vi "TestMain - Log - TDMS v2.vi"() -> ()   [LabVIEW 2019]
uses:
  <vilib>/myRIO/Instrument Drivers/Onboard IO/I2C/typedefs/I2C User Configuration.ctl
  <vilib>/myRIO/Instrument Drivers/Onboard IO/I2C/typedefs/I2C Transfer Rate.ctl
  <vilib>/Platform/TimedLoop/XDataNode/timing_clust.ctl
  <vilib>/Platform/TimedLoop/XDataNode/nitl_modes.ctl
  <vilib>/Platform/TimedLoop/XDataNode/wakeup.ctl
  <vilib>/userdefined/High Color/nirio_resource_hc.ctl
  <vilib>/myRIO/Instrument Drivers/Onboard IO/PWM/typedefs/PWM Reference.ctl
  <vilib>/myRIO/Common/Instrument Driver Framework/Utilities/typedefs/myRIO Generic Hardware Reference.ctl
  <vilib>/myRIO/Common/Instrument Driver Framework/Utilities/typedefs/Hardware Version Enum.ctl
  <vilib>/myRIO/Common/Instrument Driver Framework/Utilities/typedefs/myRIO v1.0 Reference.ctl
  <vilib>/myRIO/Common/Instrument Driver Framework/Utilities/typedefs/Generic FPGA Reference.ctl
  <vilib>/myRIO/Common/Instrument Driver Framework/myRIO v1.0/PWM/typedefs/PWM Channels Enum.ctl
  <vilib>/myRIO/Instrument Drivers/Onboard IO/PWM/typedefs/PWM Configuration.ctl
  <vilib>/myRIO/Instrument Drivers/Onboard IO/DIO/typedefs/DIO Reference.ctl
  <vilib>/myRIO/Common/Instrument Driver Framework/myRIO v1.0/DIO/typedefs/DIO Channels List.ctl
  <vilib>/myRIO/Common/Instrument Driver Framework/myRIO v1.0/DIO/typedefs/DIO Channels Enum.ctl
  <vilib>/myRIO/Common/Instrument Driver Framework/Utilities/vis/Is FPGA Ref Available.vi
  <vilib>/myRIO/Common/Instrument Driver Framework/myRIO v1.0/PWM/vis/myRIO v1.1 Open PWM.vi
  <vilib>/myRIO/Instrument Drivers/Onboard IO/PWM/vis/Set Duty Cycle and Frequency.vi
  <vilib>/myRIO/Common/Instrument Driver Framework/myRIO v1.0/DIO/vis/myRIO v1.1 Open DIO.vi
  <extravilib>/ChannelInstances/Tag-bool/Write With Abort.vi
  <extravilib>/ChannelInstances/Tag-bool/Read With Abort.vi
  <vilib>/myRIO/Common/Instrument Driver Framework/myRIO v1.0/I2C/vis/myRIO v1.0 Close I2C.vi
  <vilib>/myRIO/Common/Instrument Driver Framework/Utilities/vis/Validate Channels.vi
  <vilib>/myRIO/Common/Instrument Driver Framework/myRIO v1.0/PWM/vis/myRIO v1.0 Reserve PWM.vi
  <vilib>/myRIO/Common/Instrument Driver Framework/myRIO v1.0/DIO/vis/myRIO v1.0 Reserve DIO.vi
  <vilib>/myRIO/Common/Instrument Driver Framework/myRIO v1.0/UART/vis/myRIO v1.0 Close UART.vi
  <vilib>/myRIO/Common/Instrument Driver Framework/myRIO v1.0/I2C/vis/myRIO v1.0 Unreserve I2C.vi
  <vilib>/myRIO/Common/Instrument Driver Framework/myRIO v1.0/PWM/vis/myRIO v1.0 Build MUX Configuration PWM.vi
  <vilib>/myRIO/Common/Instrument Driver Framework/myRIO v1.0/Resource Manager/vis/myRIO v1.0 Reserve Channel List.vi
  <vilib>/myRIO/Common/Instrument Driver Framework/myRIO v1.0/DIO/vis/myRIO v1.0 Build MUX Configuration DIO.vi
  <vilib>/myRIO/Common/Instrument Driver Framework/myRIO v1.0/I2C/vis/myRIO v1.0 Build MUX Configuration I2C.vi
  <vilib>/myRIO/Common/Instrument Driver Framework/myRIO v1.0/Resource Manager/vis/myRIO v1.0 Unreserve Channel List.vi
  <vilib>/myRIO/Common/Instrument Driver Framework/myRIO v1.0/Resource Manager/vis/myRIO v1.0 Create Configuration List.vi
  <vilib>/myRIO/Common/Instrument Driver Framework/myRIO v1.0/Resource Manager/vis/myRIO v1.0 Reserve Channel.vi
  <vilib>/myRIO/Common/Instrument Driver Framework/myRIO v1.0/Resource Manager/vis/myRIO v1.0 Unreserve Channel.vi
  <vilib>/myRIO/Common/Instrument Driver Framework/myRIO v1.0/Resource Manager/vis/myRIO v1.0 Build Mutex Name.vi
  <vilib>/FPGAPlugInAG/myRIO-1900/niLvFpga_Open_myRIO-1900.vi
  <vilib>/rvi/interface/common/dynamic/niFpgaDynamicAddResources.vi
  <vilib>/Utility/error.llb/Error Cluster From Error Code.vi
  <vilib>/rvi/errors/niLvFpgaAdjustHostInterfaceError.vi
  <vilib>/myRIO/Common/Instrument Driver Framework/Utilities/vis/FPGA Ref Manager.vi
  <vilib>/myRIO/Common/Instrument Driver Framework/Utilities/vis/Ref Counter.vi
  <vilib>/FPGAPlugInAG/Dynamic/niLvFpga_Run_Dynamic.vi
  <vilib>/myRIO/Common/Instrument Driver Framework/myRIO v1.0/I2C/vis/myRIO v1.0 Configure I2C.vi
  <vilib>/myRIO/Common/Instrument Driver Framework/myRIO v1.0/I2C/vis/myRIO v1.0 Write I2C.vi
  <vilib>/Utility/VariantDataType/GetNumericInfo.vi
  <vilib>/myRIO/Common/Instrument Driver Framework/myRIO v1.0/myRIO v1.1 Open.vi
  <vilib>/myRIO/Common/Instrument Driver Framework/Utilities/vis/IO Manager.vi
  <vilib>/myRIO/Common/Instrument Driver Framework/Utilities/vis/Configuration Manager.vi
  <vilib>/myRIO/Common/Instrument Driver Framework/myRIO v1.0/Resource Manager/vis/myRIO v1.0 Configure IO.vi
  <vilib>/myRIO/Common/Instrument Driver Framework/myRIO v1.0/myRIO v1.0 Close.vi
  <vilib>/myRIO/Common/Instrument Driver Framework/myRIO v1.0/PWM/vis/myRIO v1.0 Write PWM.vi
  <vilib>/myRIO/Common/Instrument Driver Framework/myRIO v1.0/DIO/vis/myRIO v1.0 Write DIO.vi
  <vilib>/Instr/_visa.llb/VISA Configure Serial Port (Instr).vi
  <extravilib>/ChannelInstances/Tag-bool/Instantiate.vi
  <extravilib>/ChannelInstances/Tag-bool/EndpointRead.vi
  <vilib>/myRIO/Common/Instrument Driver Framework/myRIO v1.0/I2C/vis/myRIO v1.0 Read I2C.vi
  <vilib>/myRIO/Common/Instrument Driver Framework/myRIO v1.0/I2C/vis/myRIO v1.0 Shutdown I2C.vi
  <vilib>/FPGAPlugInAG/Dynamic/niLvFpga_Abort_Dynamic.vi
  <vilib>/myRIO/Common/Instrument Driver Framework/myRIO v1.0/myRIO v1.0 Reset FPGA.vi
  <vilib>/myRIO/Common/Instrument Driver Framework/myRIO v1.0/IRQ/vis/myRIO v1.0 IRQ Info FGV.vi
  <vilib>/myRIO/Common/Instrument Driver Framework/myRIO v1.0/IRQ/vis/myRIO v1.0 Timer IRQ Info FGV.vi
  <vilib>/myRIO/Common/Instrument Driver Framework/myRIO v1.0/IRQ/vis/myRIO v1.0 ISR Agent.vi
  <vilib>/myRIO/Instrument Drivers/Utilities/vis/Reset Index.vi
  <vilib>/myRIO/Common/Instrument Driver Framework/myRIO v1.0/Resource Manager/vis/myRIO v1.0 Block Write Resource Manager.vi
  <vilib>/FPGAPlugInAG/Dynamic/niLvFpga_Close_Dynamic.vi
  <extravilib>/ChannelInstances/Tag-bool/Endpoint.vi
  <vilib>/platform/TimedLoop/XDataNode/XDataNode.xnode
  <vilib>/rvi/interface/nirviOpenFPGA/nirviOpenFPGA.xnode
  Documents/Source_Distribution/AutoBike_Autumn2021_src_lvproj/home/lvuser/natinst/bin/autobike_FPGATarget_myRIO-1900Custom_zQgCF+RzkZg.lvbitx
  <vilib>/rvi/interface/nirviReadWriteControl/nirviReadWriteControl.xnode
  <vilib>/rvi/interface/nirviMethod/nirviMethod.xnode
  <vilib>/myRIO/Express VI/Onboard IO/PWM/PWM Express VI.xnode
  <vilib>/myRIO/Instrument Drivers/Onboard IO/PWM/vis/myRIO PWM Open.xnode
  <vilib>/myRIO/Express VI/Onboard IO/DO/DO Express VI.xnode
  <vilib>/myRIO/Instrument Drivers/Onboard IO/DIO/vis/myRIO DIO Open.xnode
  <vilib>/rvi/interface/nirviCloseFPGA/nirviCloseFPGA.xnode
  <vilib>/myRIO/Instrument Drivers/Utilities/Utilities.lvlib
  NiFpgaLv.dll
  <vilib>/rvi/interface/Simulation/niFpgaSimulationCallBeginRW.vi
  <vilib>/Platform/TimedLoop/XDataNode/XDNodeRunTimeDep.lvlib
  <extravilib>/ChannelInstances/Tag-bool.lvlib
  <vilib>/myRIO/Instrument Drivers/Onboard IO/I2C/I2C.lvlib
  <vilib>/myRIO/Instrument Drivers/Onboard IO/DIO/DIO.lvlib
  <vilib>/myRIO/Instrument Drivers/Onboard IO/PWM/PWM.lvlib
panel:
  out "Raw output from GPS":string
  in  "Organised Output from the GPS":T1(tab)
  out "GPGSV":string
  out "number of message":string
  out "msg1":string
  out "Satelite in view":string
  in  "Satelite_id/elevation/azimuth/SNR 17":enum32{"Msg 1", "Msg 2", "Msg 3", "Msg 4"}(tab)
  out "Satelite_id/elevation/azimuth/SNR":string[](array[string])
  out "Satelite_id/elevation/azimuth/SNR 2":string[](array[string])
  out "Satelite_id/elevation/azimuth/SNR 3":string[](array[string])
  out "Satelite_id/elevation/azimuth/SNR 4":string[](array[string])
  out "Signal ID / Check sum":string[](array[string])
  out "Signal ID / Check sum 2":string[](array[string])
  out "Satelite_id/elevation/azimuth/SNR 8":string[](array[string])
  out "Satelite_id/elevation/azimuth/SNR 7":string[](array[string])
  out "Satelite_id/elevation/azimuth/SNR 6":string[](array[string])
  out "Satelite_id/elevation/azimuth/SNR 5":string[](array[string])
  out "Signal ID / Check sum 3":string[](array[string])
  out "Satelite_id/elevation/azimuth/SNR 12":string[](array[string])
  out "Satelite_id/elevation/azimuth/SNR 11":string[](array[string])
  out "Satelite_id/elevation/azimuth/SNR 10":string[](array[string])
  out "Satelite_id/elevation/azimuth/SNR 9":string[](array[string])
  out "Signal ID / Check sum 4":string[](array[string])
  out "Satelite_id/elevation/azimuth/SNR 16":string[](array[string])
  out "Satelite_id/elevation/azimuth/SNR 15":string[](array[string])
  out "Satelite_id/elevation/azimuth/SNR 14":string[](array[string])
  out "Satelite_id/elevation/azimuth/SNR 13":string[](array[string])
  out "GLGSV 2":string
  out "number of message 2":string
  out "msg1 2":string
  out "Satelite in view 2":string
  in  "Satelite_id/elevation/azimuth/SNR 34":enum32{"Msg 1", "Msg 2", "Msg 3", "Msg 4"}(tab)
  out "Satelite_id/elevation/azimuth/SNR 21":string[](array[string])
  out "Satelite_id/elevation/azimuth/SNR 20":string[](array[string])
  out "Satelite_id/elevation/azimuth/SNR 19":string[](array[string])
  out "Satelite_id/elevation/azimuth/SNR 18":string[](array[string])
  out "Signal ID / Check sum 5":string[](array[string])
  out "Signal ID / Check sum 6":string[](array[string])
  out "Satelite_id/elevation/azimuth/SNR 25":string[](array[string])
  out "Satelite_id/elevation/azimuth/SNR 22":string[](array[string])
  out "Satelite_id/elevation/azimuth/SNR 23":string[](array[string])
  out "Satelite_id/elevation/azimuth/SNR 24":string[](array[string])
  out "Signal ID / Check sum 7":string[](array[string])
  out "Satelite_id/elevation/azimuth/SNR 29":string[](array[string])
  out "Satelite_id/elevation/azimuth/SNR 26":string[](array[string])
  out "Satelite_id/elevation/azimuth/SNR 27":string[](array[string])
  out "Satelite_id/elevation/azimuth/SNR 28":string[](array[string])
  out "Signal ID / Check sum 8":string[](array[string])
  out "Satelite_id/elevation/azimuth/SNR 33":string[](array[string])
  out "Satelite_id/elevation/azimuth/SNR 30":string[](array[string])
  out "Satelite_id/elevation/azimuth/SNR 31":string[](array[string])
  out "Satelite_id/elevation/azimuth/SNR 32":string[](array[string])
  out "GAGSV 3":string
  out "number of message 3":string
  out "msg1 3":string
  out "Satelite in view 3":string
  in  "Satelite_id/elevation/azimuth/SNR 51":enum32{"Msg 1", "Msg 2", "Msg 3", "Msg 4"}(tab)
  out "Satelite_id/elevation/azimuth/SNR 38":string[](array[string])
  out "Satelite_id/elevation/azimuth/SNR 37":string[](array[string])
  out "Satelite_id/elevation/azimuth/SNR 36":string[](array[string])
  out "Satelite_id/elevation/azimuth/SNR 35":string[](array[string])
  out "Signal ID / Check sum 9":string[](array[string])
  out "Signal ID / Check sum 10":string[](array[string])
  out "Satelite_id/elevation/azimuth/SNR 42":string[](array[string])
  out "Satelite_id/elevation/azimuth/SNR 39":string[](array[string])
  out "Satelite_id/elevation/azimuth/SNR 40":string[](array[string])
  out "Satelite_id/elevation/azimuth/SNR 41":string[](array[string])
  out "Signal ID / Check sum 11":string[](array[string])
  out "Satelite_id/elevation/azimuth/SNR 46":string[](array[string])
  out "Satelite_id/elevation/azimuth/SNR 43":string[](array[string])
  out "Satelite_id/elevation/azimuth/SNR 44":string[](array[string])
  out "Satelite_id/elevation/azimuth/SNR 45":string[](array[string])
  out "Signal ID / Check sum 12":string[](array[string])
  out "Satelite_id/elevation/azimuth/SNR 50":string[](array[string])
  out "Satelite_id/elevation/azimuth/SNR 47":string[](array[string])
  out "Satelite_id/elevation/azimuth/SNR 48":string[](array[string])
  out "Satelite_id/elevation/azimuth/SNR 49":string[](array[string])
  out "GBGSV 4":string
  out "number of message 4":string
  out "msg1 4":string
  out "Satelite in view 4":string
  in  "Satelite_id/elevation/azimuth/SNR 68":enum32{"Msg 1", "Msg 2", "Msg 3", "Msg 4"}(tab)
  out "Satelite_id/elevation/azimuth/SNR 55":string[](array[string])
  out "Satelite_id/elevation/azimuth/SNR 54":string[](array[string])
  out "Satelite_id/elevation/azimuth/SNR 53":string[](array[string])
  out "Satelite_id/elevation/azimuth/SNR 52":string[](array[string])
  out "Signal ID / Check sum 13":string[](array[string])
  out "Signal ID / Check sum 14":string[](array[string])
  out "Satelite_id/elevation/azimuth/SNR 59":string[](array[string])
  out "Satelite_id/elevation/azimuth/SNR 56":string[](array[string])
  out "Satelite_id/elevation/azimuth/SNR 57":string[](array[string])
  out "Satelite_id/elevation/azimuth/SNR 58":string[](array[string])
  out "Signal ID / Check sum 15":string[](array[string])
  out "Satelite_id/elevation/azimuth/SNR 63":string[](array[string])
  out "Satelite_id/elevation/azimuth/SNR 60":string[](array[string])
  out "Satelite_id/elevation/azimuth/SNR 61":string[](array[string])
  out "Satelite_id/elevation/azimuth/SNR 62":string[](array[string])
  out "Signal ID / Check sum 16":string[](array[string])
  out "Satelite_id/elevation/azimuth/SNR 67":string[](array[string])
  out "Satelite_id/elevation/azimuth/SNR 64":string[](array[string])
  out "Satelite_id/elevation/azimuth/SNR 65":string[](array[string])
  out "Satelite_id/elevation/azimuth/SNR 66":string[](array[string])
  out "UTC Time":string
  out "N/S":string
  out "Long":string
  out "Mode":string
  out "Status":string
  out "Lat":string
  out "Course over Ground [Degrees]":string
  out "date[ddmmyy]":string
  out "E/W":string
  out "Speed over ground[knot]":string
  out "xxRMC":string
  out "NavStatus":string
  out "Checksum":string
  out "Carriage return":string
  out "Lat 2":string
  out "NS":string
  out "GLL":string
  out "Long 3":string
  out "EW":string
  out "Time":string
  out "Status 2":string
  out "Positioning mod":string
  out "Check sum":string
  out "Carriage return 2":string
  out "VTG":string
  out "Course over Ground":string
  out "Reference":string
  out "Course over Ground (Magnetic)":string
  out "Reference2":string
  out "Speedover Ground (knots)":string
  out "Units1":string
  out "Speed over ground kph":string
  out "Units 2":string
  out "Position Mode 2":string
  out "Check sum 2":string
  out "GGA 3":string
  out "UTC time":string
  out "Lat 3":string
  out "NS 2":string
  out "Long 2":string
  out "EW 2":string
  out "Pos_indicator":string
  out "Number of Satelite_used":string
  out "hdop":string
  out "msl_altitude":string
  out "altitude_units":string
  out "geoidal_Seperation":string
  out "Separation unit":string
  out "age of Diff corr":string
  out "diffStating":string
  out "Checksum 2":string
  out "GSA":string
  out "Operation Mode":string
  out "Navigation mode":string
  out "satelite used channel 1":string
  out "satelite used channel 3":string
  out "satelite used channel 4":string
  out "satelite used channel 5":string
  out "satelite used channel 6":string
  out "satelite used channel 7":string
  out "satelite used channel 8":string
  out "satelite used channel 9":string
  out "satelite used channel 10":string
  out "satelite used channel 11":string
  out "satelite used channel 12":string
  out "pdop":string
  out "hdop 2":string
  out "vdop":string
  out "System ID":string
  out "Checksum 3":string
  out "satelite used channel 2":string
  in  "Name of the Logging file":string="Logging.tdms"
  out "Path to the Logg file":path
  out "Combined duration time (us)":i64
  in  "Loop durations":T2(tab)
  out "IMU Data gathering duration(us)":i64(graph)
  out "Hall data gathering duration(us)":i64(graph)
  out "Encoder data gathering duration(us)":i64(graph)
  out "Steering Motor Sending/updating value duration(us)":i64(graph)
  out "E-Stop loop duration (us)":i64(graph)
  out "GPS loop duration (us)":i64(graph)
  in  "Duty cycle":dbl(slide)=0.5 step=0.01 scale=0.1..0.9
  in  "GO":bool
  out "E-Stop":bool
  in  "E-stop":bool
  in  "IMU":bool
  out "IMU Acc Chart":cluster{dbl, dbl, dbl}(graph)
  out "IMU Gyro Chart":cluster{dbl, dbl, dbl}(graph)
  out "Encoder Position (Counts)":i32
  out "Encoder Acceleration (Counts/Interval)":i32
  out "Encoder Velocity (Counts/Interval)":i32
  in  "Encoder":bool
  in  "Encoder Position Reset":bool
  out "Hall Period":u32
  in  "Hall":bool
  out "Hall Detection":bool
  # "Signal ID / Check sum"
  # "Signal ID / Check sum"
  # "Signal ID / Check sum"
  # "Signal ID / Check sum"
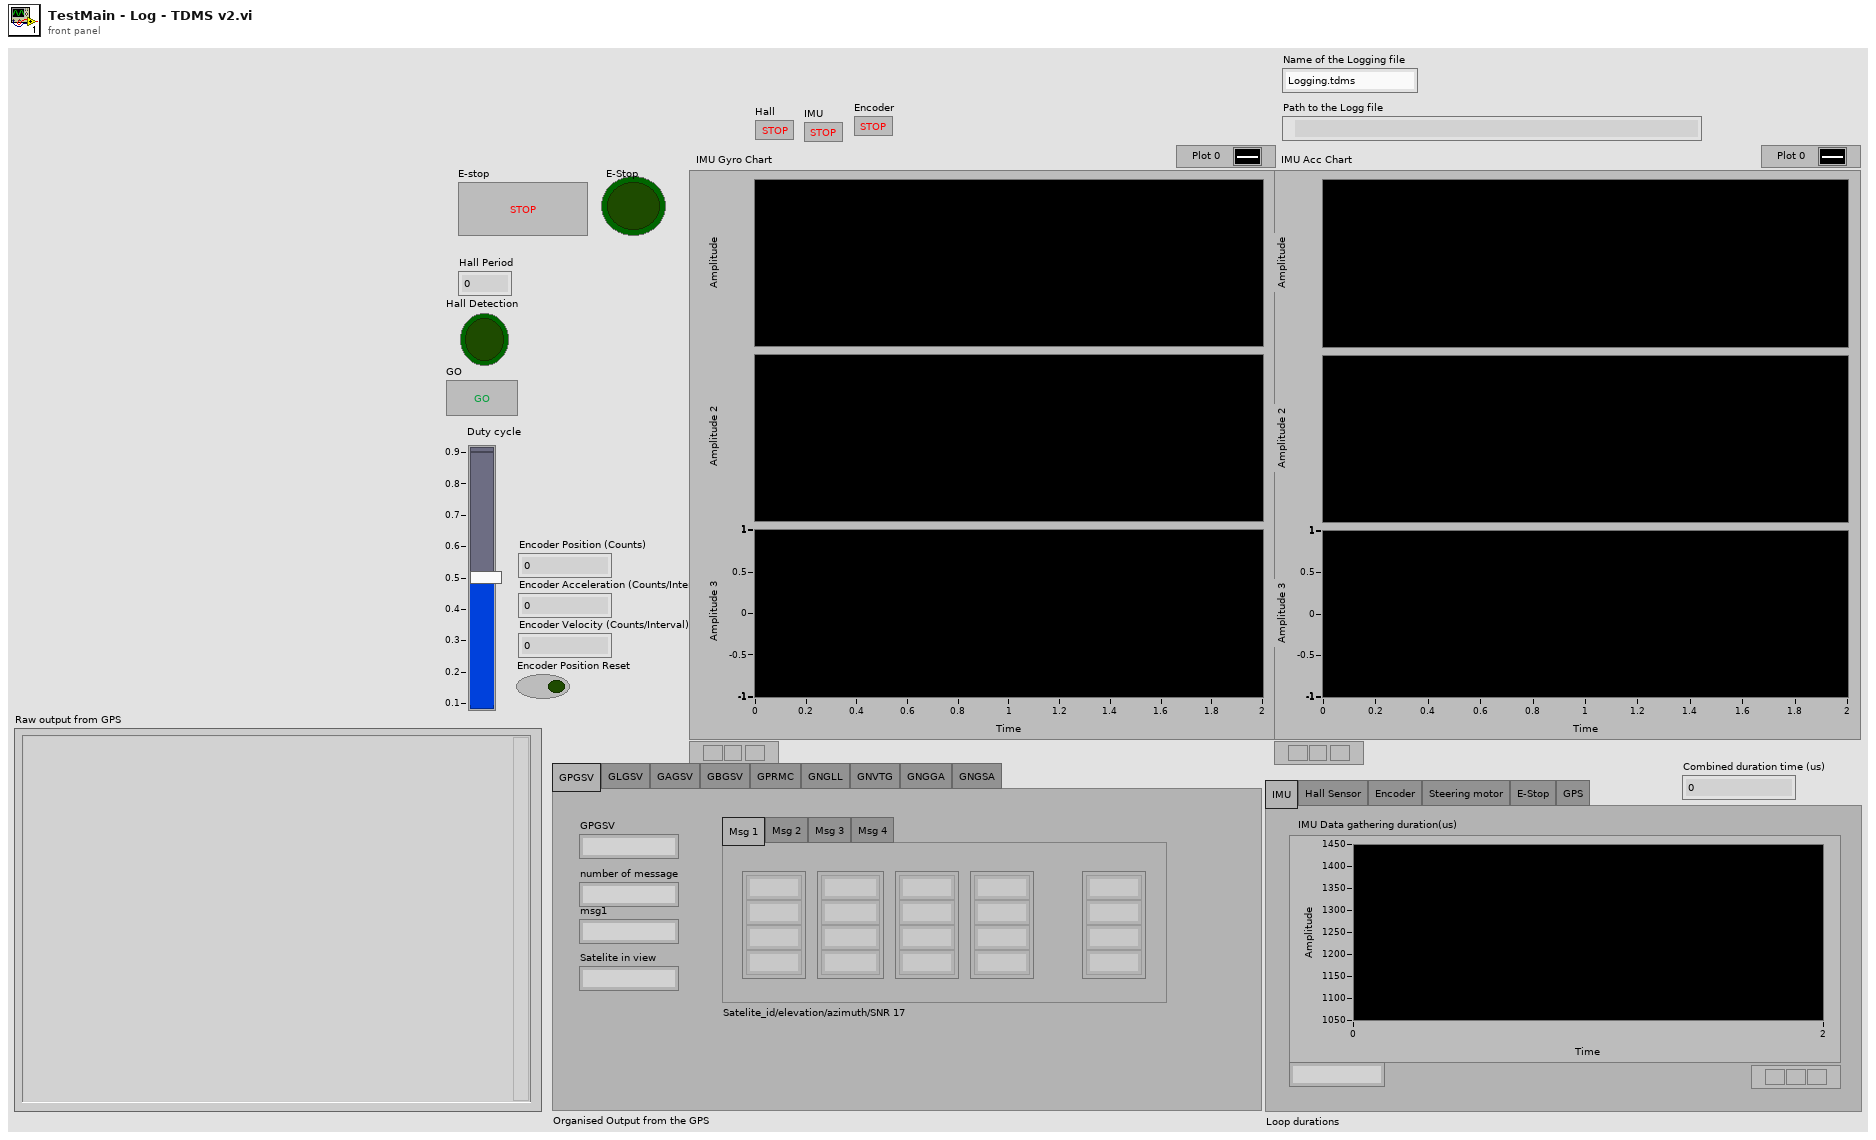
[diagram p1: front panel]
types:
  T1 = enum32{"GPGSV", "GLGSV", "GAGSV", "GBGSV", "GPRMC", "GNGLL", "GNVTG", "GNGGA", "GNGSA"}
  T2 = enum32{"IMU", "Hall Sensor", "Encoder", "Steering motor", "E-Stop", "GPS"}
  T3 = typedef "I2C.lvlib/I2C User Configuration.ctl" = cluster{"I2C Transfer Rate":T4}
  T4 = typedef "I2C.lvlib/I2C Transfer Rate.ctl" = enum16{"Standard mode (100 kbps)", "Fast mode (400 kbps)"}
  T5 = enum16{"open", "open or create", "create or replace", "create", "open (read-only)"}
  T6 = typedef "nirio_resource_hc.ctl" = tag
  T7 = typedef "I2C.lvlib/I2C Reference.ctl" = cluster{"myRIO Reference":T8, "I2C Channels Enum":T12, "I2C Configuration":T13}
  T8 = typedef "myRIO Generic Hardware Reference.ctl" = cluster{"myRIO Model":T9, "myRIO Hardware Reference":T10}
  T9 = typedef "Hardware Version Enum.ctl" = enum16{"Unknown", "myRIO-1900", "myRIO-1950", "roboRIO", "NI ELVIS RIO CM", "ELVIS III"}
  T10 = typedef "myRIO v1.0 Reference.ctl" = cluster{"Generic FPGA Reference":T11, "Allow multiple opens":bool}
  T11 = typedef "Generic FPGA Reference.ctl" = refnum<k20>
  T12 = typedef "I2C Channels Enum.ctl" = enum16{"Not Connected", "A/I2C", "B/I2C", "I2C/I2C"}
  T13 = typedef "I2C.lvlib/I2C Configuration.ctl" = cluster{"I2C Transfer Rate":T4}
  T14 = typedef "XDNodeRunTimeDep.lvlib/timing_clust.ctl" = cluster{"Expected End [f-1]":u64, "Actual End [f-1]":u64, "Finished Late? [f-1]":bool, "Expected End [i-1]":u64, "Actual End [i-1]":u64, "Finished Late? [i-1]":bool, "Expected Start [i]":u64, "Actual Start [i]":u64, "Expected Start [f]":u64, "Actual Start [f]":u64, "Source Name":string, "Structure Name":string, "Period":i64, "Deadline":i64, "Offset":i64, "Start":i64, "Priority":i32, "Timeout":i32, "Mode":T15, "Wakeup Reason":T16, "Error":errorcluster, "Source Type":string, "Secondary Source Type":string, "Global End Time":u64, "Global Start Time":u64, "Frame Duration":u64, "Iteration Duration":u64, "Assigned CPU":i32, "I/O Scan Engine Mode":u32}
  T15 = typedef "XDNodeRunTimeDep.lvlib/nitl_modes.ctl" = enum32{"No Change", "Process missed periods, maintain original phase", "Discard missed periods, maintain original phase", "Process missed periods, ignore original phase", "Discard missed periods, ignore original phase"}
  T16 = typedef "XDNodeRunTimeDep.lvlib/wakeup.ctl" = enum32{"Normal", "Aborted", "Asynchronous wakeup", "Timing source error", "Timed loop error", "Timeout"}
  T17 = typedef "PWM.lvlib/PWM Reference.ctl" = cluster{"myRIO Reference":T8, "PWM Channels Enum":T18, "PWM Configuration":T19}
  T18 = typedef "PWM Channels Enum.ctl" = enum16{"Not Connected", "C/PWM0", "C/PWM1", "A/PWM0", "A/PWM1", "A/PWM2", "A/PWM3", "A/PWM4", "A/PWM5", "A/PWM6", "A/PWM7", "A/PWM8", "A/PWM9", "A/PWM10", "A/PWM11", "A/PWM12", "A/PWM13", "A/PWM14", "A/PWM15", "A/PWM16", "A/PWM17", "A/PWM18", "A/PWM19", "B/PWM0", "B/PWM1", "B/PWM2", "B/PWM3", "B/PWM4", "B/PWM5", "B/PWM6", "B/PWM7", "B/PWM8", "B/PWM9", "B/PWM10", "B/PWM11", "B/PWM12", "B/PWM13", "B/PWM14", "B/PWM15", "B/PWM16", "B/PWM17", "B/PWM18", "B/PWM19", "PWM/PWM0", "PWM/PWM1", "PWM/PWM2", "PWM/PWM3", "PWM/PWM4", "PWM/PWM5", "PWM/PWM6", "PWM/PWM7", "PWM/PWM8", "PWM/PWM9"}
  T19 = typedef "PWM.lvlib/PWM Configuration.ctl" = cluster{"Frequency":dbl, "Duty Cycle":dbl}
  T20 = typedef "DIO.lvlib/DIO Reference.ctl" = cluster{"myRIO Reference":T8, "DIO Channels List":T21}
  T21 = typedef "DIO Channels List.ctl" = T22[]
  T22 = typedef "DIO Channels Enum.ctl" = enum16{"Not Connected", "C/DIO0", "C/DIO1", "C/DIO2", "C/DIO3", "C/DIO4", "C/DIO5", "C/DIO6", "C/DIO7", "A/DIO0", "A/DIO1", "A/DIO2", "A/DIO3", "A/DIO4", "A/DIO5", "A/DIO6", "A/DIO7", "A/DIO8", "A/DIO9", "A/DIO10", "A/DIO11", "A/DIO12", "A/DIO13", "A/DIO14", "A/DIO15", "A/DIO16", "A/DIO17", "A/DIO18", "A/DIO19", "B/DIO0", "B/DIO1", "B/DIO2", "B/DIO3", "B/DIO4", "B/DIO5", "B/DIO6", "B/DIO7", "B/DIO8", "B/DIO9", "B/DIO10", "B/DIO11", "B/DIO12", "B/DIO13", "B/DIO14", "B/DIO15", "B/DIO16", "B/DIO17", "B/DIO18", "B/DIO19", "LED0", "LED1", "LED2", "LED3", "Button0", "DIO/DIO0", "DIO/DIO1", "DIO/DIO2", "DIO/DIO3", "DIO/DIO4", "DIO/DIO5", "DIO/DIO6", "DIO/DIO7", "DIO/DIO8", "DIO/DIO9", "SPI/CS0", "SPI/CS1", "SPI/CS2", "SPI/CS3", "LED RADIO (Green)", "LED RADIO (Red)", "LED COMM (Green)", "LED COMM (Red)", "LED MODE (Green)", "LED MODE (Red)"}
  T23 = typedef "Tag-bool.lvlib/))Channel.ctl" = refnum<queue>
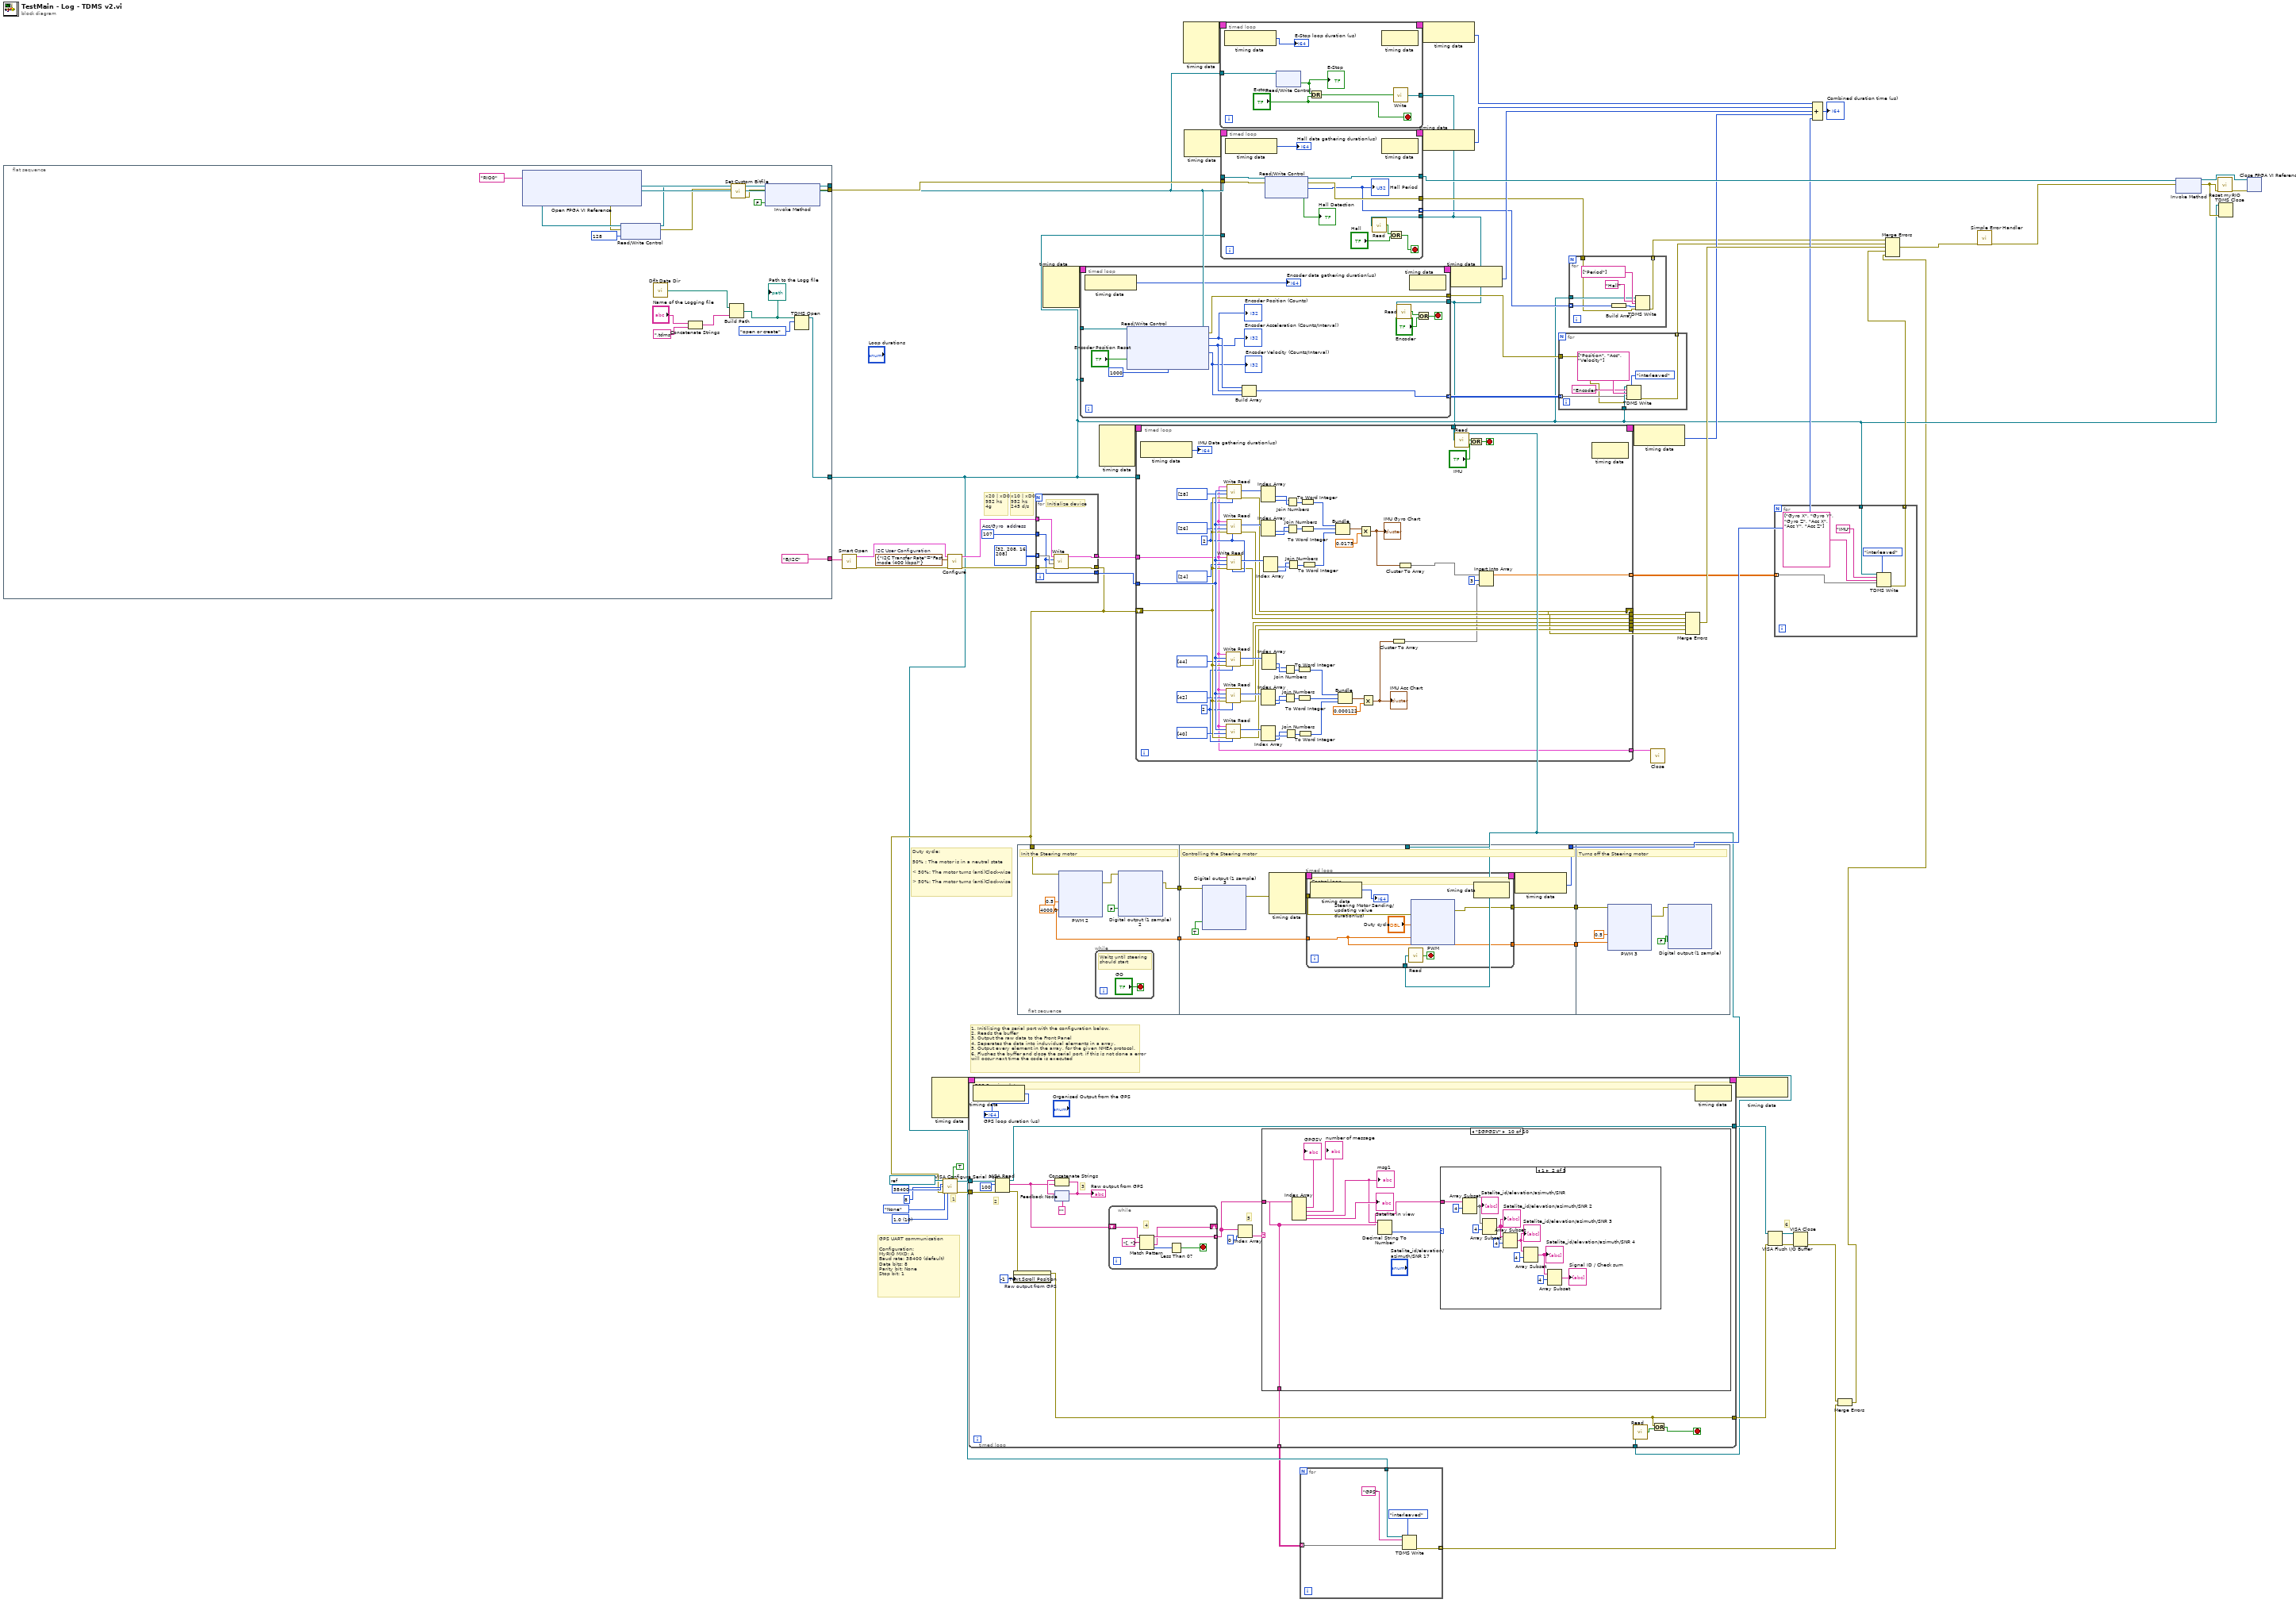
[diagram p0: block diagram]
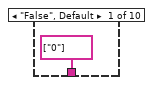
[diagram p2: hidden frame]
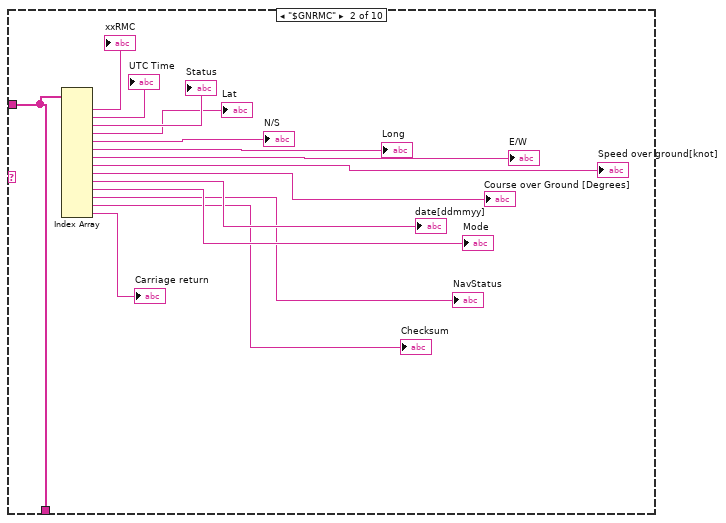
[diagram p3: hidden frame]
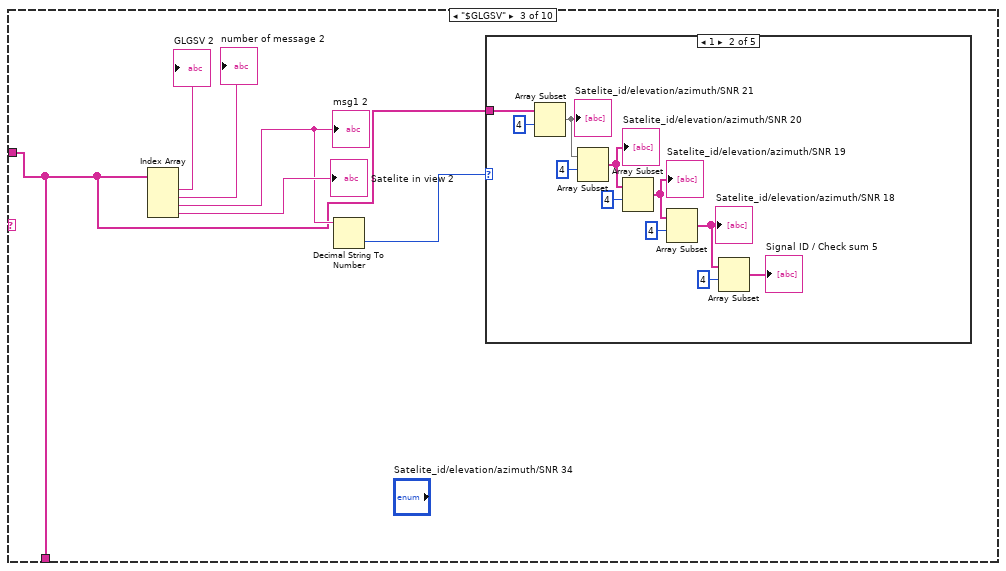
[diagram p4: hidden frame]
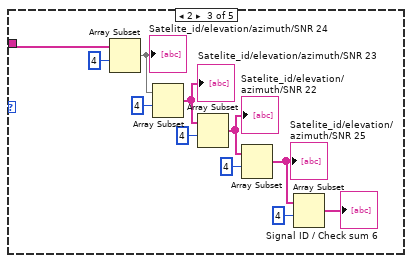
[diagram p6: hidden frame]
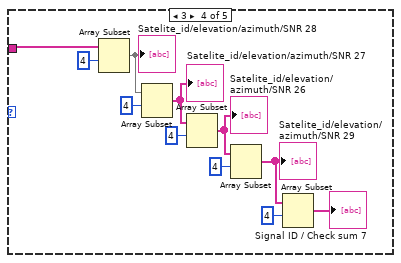
[diagram p7: hidden frame]
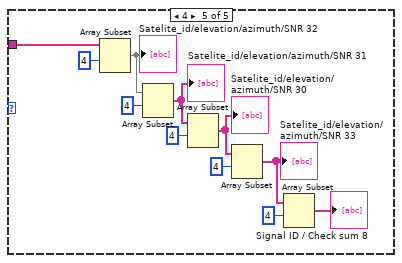
[diagram p8: hidden frame]
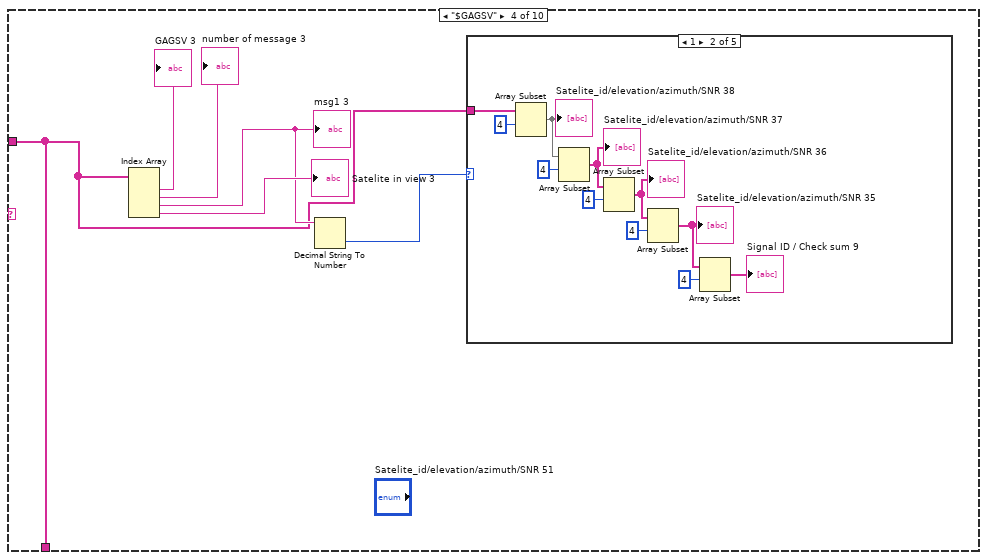
[diagram p9: hidden frame]
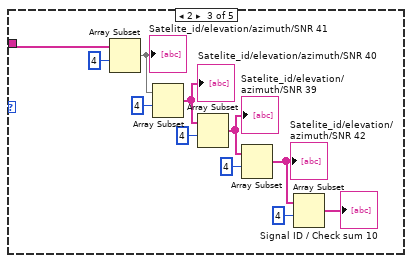
[diagram p11: hidden frame]
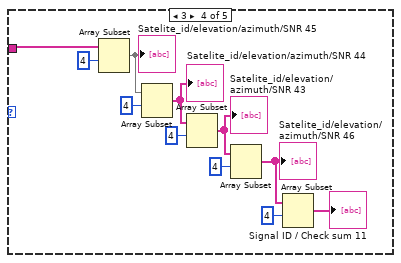
[diagram p12: hidden frame]
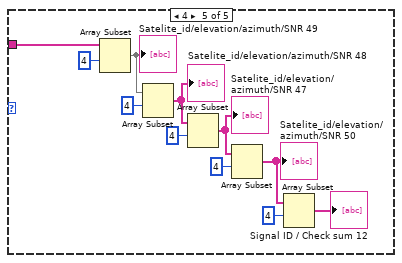
[diagram p13: hidden frame]
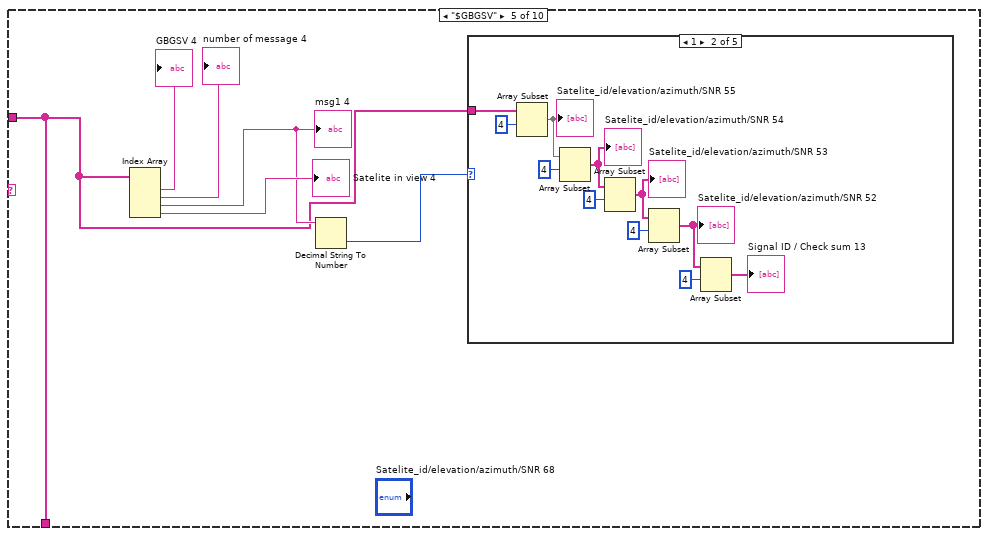
[diagram p14: hidden frame]
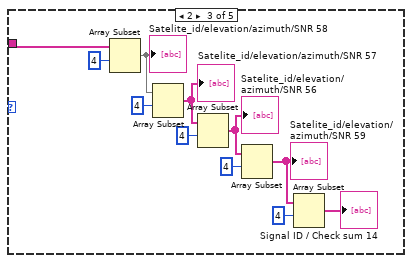
[diagram p16: hidden frame]
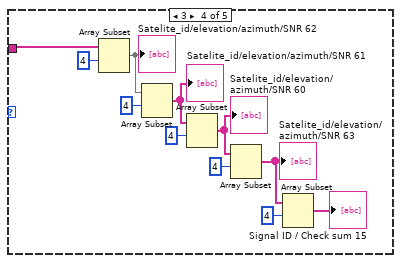
[diagram p17: hidden frame]
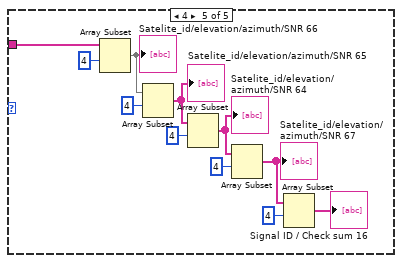
[diagram p18: hidden frame]
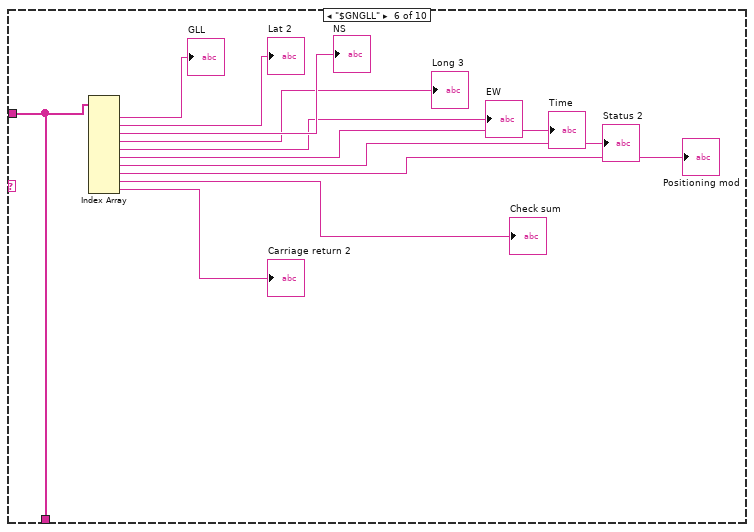
[diagram p19: hidden frame]
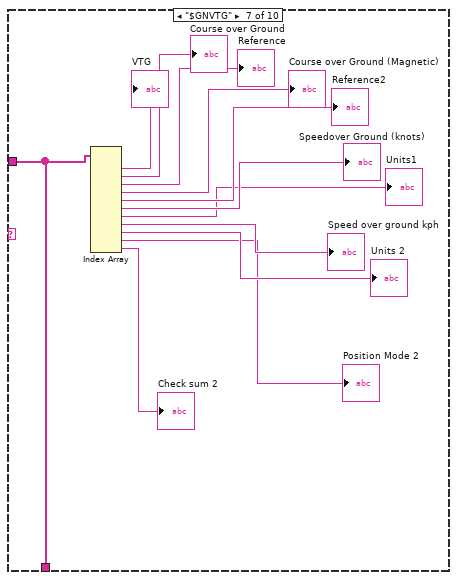
[diagram p20: hidden frame]
diagram:
  w15 = u16 10 items=["1.0"=10, "1.5"=15, "2.0"=20] ("stop bits (10: 1 bit)")
  w48 = u8 107  # Acc/Gyro  address
  w51 = T3 {"I2C Transfer Rate"=enum."Fast mode (400 kbps)"}  # I2C User Configuration
  # "6"
  # "1"
  # "1. Initilizing the serial port with the configuration below.\n2. Reads the buffer\n3. Output the raw data to the Front Panel\n4. Seperates the data into induvidual elements in a array.\n5. Output every element in the array, for the given NMEA protocol.\n6. Flushes the buffer and close the serial port, if this is not done a error will occur next time the code is executed"
  # "GPS UART communication\n\nConfiguration:\nMyRIO MXD: A\nBaud rate: 38400 (default)\nData bits: 8\nParity bit: None\nStop bit: 1"
  # "Duty cycle:\n\n50% : The motor is in a neutral state\n\n< 50%: The motor turns (anti)Clock-wise\n\n> 50%: The motor turns (anti)Clock-wise"
  # "x20 | xD0\n952 hz\n4g"
  # "x10 | xD0\n952 hz\n245 d/s"
  n1 = flat-sequence {
    tunnel: [w92] -> w61
    tunnel: [tag "B/I2C" ("I2C I/O")] -> w44
    tunnel: [w90] -> w40
    tunnel: [w80] -> w6
    frame #0 {
      n2 = xnode "Open FPGA VI Reference"("resource name"=T6 "RIO0" ("Resource name")) -> ("FPGA VI Reference Out"=w82:refnum<k20>, "error out"=w81:errorcluster)  [unwired: 1 in]
      n3 = xnode "Read/Write Control"("FPGA VI Reference In"=w82, "error in"=w81, "SYS.SELECTB"=u8 128) -> ("FPGA VI Reference Out"=w86:refnum<k20>, "error out"=w85:errorcluster)
      n4 = call <vilib>:"Dflt Data Dir.vi"() -> ("App:Default Data Directory"=w79:path)
      n5 = Concatenate Strings("Name of the Logging file", ".tdms" ("string")) -> (w74:string)
      n6 = Build Path(base path=w79, name or relative path=w74) -> (appended path=w78:path)
      "Path to the Logg file" <- w78
      n7 = call <vilib>:"Set Custom Bitfile.vi"("error in (no error)"=w85, "Custom FPGA Reference In"=w86) -> ("error out"=w87:errorcluster, "Custom FPGA Reference Out"=w89:refnum<k20>)  [unwired: 8 in]
      n8 = xnode "Invoke Method"("FPGA VI Reference In"=w89, "error in"=w87, "Wait Until Done (F)"=FALSE) -> ("FPGA VI Reference Out"=w90:refnum<k20>, "error out"=w92:errorcluster)
      n9 = TDMS Open(10:T5."open or create" ("operation (0:open)"), 11:w78) -> (3:w80:refnum<k34>)  [unwired: 5 in, 1 out]
    }
  }
  n10 = call <vilib>:"Smart Open.vi"("Channel Name"=w44) -> ("error out"=w49:errorcluster, "I2C Ref Out"=w50:T7)  [unwired: 9 in]
  n11 = node-c288() -> (w22:T14)  [unwired: 4 in]
  n12 = call <vilib>:"Configure.vi"("error in (no error)"=w49, "I2C User Configuration"=w51, "I2C Ref In"=w50) -> ("error out"=w45:errorcluster, "I2C Ref Out"=w46:T7)  [unwired: 7 in]
  n13 = flat-sequence {
    tunnel: [w97] -> w65
    tunnel: w8 -> [w95]
    tunnel: [w94] -> w64
    tunnel: w4 -> [w179]
    tunnel: w65 -> [w177]
    tunnel: w64 -> [w176]
    tunnel: [w175] -> w63
    tunnel: [w174] -> w62
    tunnel: [w171] -> w36
    tunnel: w63 -> [w266]
    tunnel: w62 -> [w265]
    frame #0 {
      w94 = 4000.0 ("Frequency [Hz]")
      # "Init the Steering motor"
      n14 = xnode "PWM 2"("Duty Cycle"=0.5, "Frequency [Hz]"=w94, "error in (no error)"=w95) -> ("error out"=w98:errorcluster)
      n15 = while {
        stop <- "GO" stop-if-true
        # "Waits until steering should start"
      }
      n16 = xnode "Digital output (1 sample) 2"("B/DIO4 (Pin 19)"=FALSE ("B/DIO1 (Pin 13)"), "error in (no error)"=w98) -> ("error out"=w97:errorcluster)
    }
    frame #1 {
      # "Controlling the Steering motor"
      n17 = xnode "Digital output (1 sample) 3"("B/DIO4 (Pin 19)"=TRUE ("B/DIO1 (Pin 13)"), "error in (no error)"=w177) -> ("error out"=w178:errorcluster)
      n18 = node-c288() -> (w173:T14)  [unwired: 4 in]
      n19 = timed-loop {
        tunnel: w179 -> [w184]
        tunnel: w178 -> [w183]
        tunnel: w176 -> [w182]
        tunnel: [w182] -> w175
        tunnel: [w181] -> w174
        timing: w173 -> [_]
        timing-out: [_] -> w172
        stop <- w185 stop-if-true
        # "Control loop"
        n20 = node-c288() -> (→"Steering Motor Sending/updating value duration(us)":i64)  [unwired: 1 in]
        n21 = call <extravilib>:"Read.vi"("channel"=w184) -> ("element"=w185:bool)  [unwired: 1 in, 1 out]
        n22 = xnode "PWM"("Duty Cycle"="Duty cycle", "Frequency [Hz]"=w182, "error in (no error)"=w183) -> ("error out"=w181:errorcluster)
        n23 = node-c288() -> ()  [unwired: 1 in, 1 out]
      }
      n24 = node-c288(w172) -> (w171:i64)
    }
    frame #2 {
      # "Turns off the Steering motor"
      n25 = xnode "PWM 3"("Duty Cycle"=0.5, "Frequency [Hz]"=w266, "error in (no error)"=w265) -> ("error out"=w264:errorcluster)
      n26 = xnode "Digital output (1 sample)"("B/DIO4 (Pin 19)"=FALSE ("B/DIO1 (Pin 13)"), "error in (no error)"=w264) -> ()  [unwired: 1 out]
    }
  }
  n27 = for {
    tunnel: [w338] -> w8
    tunnel: [w339] -> w33
    tunnel: [w340] -> w32
    tunnel: u8[][] [[32, 208], [16, 208]] ("Bytes to Write") -> [w341] mode=indexing
    tunnel: w46 -> [w343]
    tunnel: w45 -> [w342]
    tunnel: w48 -> [w340]
    # "Initialize device"
    n28 = call <vilib>:"Write.vi"("error in (no error)"=w342, "Bytes to Write"=w341, "Slave Address (7-bit)"=w340, "I2C Ref In"=w343) -> ("error out"=w338:errorcluster, "I2C Ref Out"=w339:T7)  [unwired: 6 in]
  }
  n29 = call-poly "VISA Configure Serial Port"("VISA resource name"=refnum<visa-resource-name> "ASRL1::INSTR", "Enable Termination\nChar (T)"=TRUE ("Enable Termination\nChar (T)"), "baud rate (9600)"=u32 38400, "data bits (8)"=u16 8, "parity (0:none)"=enum16{"None", "Odd", "Even", "Mark", "Space"}."None", "error in (no error)"=w8, "stop bits (10: 1 bit)"=w15) -> ("VISA resource name out"=w11:refnum<visa-resource-name>, "error out"=w10:errorcluster)  [unwired: 7 in]
  n30 = node-c288() -> (w71:T14)  [unwired: 4 in]
  n31 = node-c288() -> (w69:T14)  [unwired: 4 in]
  n32 = node-c288() -> (w67:T14)  [unwired: 4 in]
  n33 = node-c288() -> (w73:T14)  [unwired: 2 in]
  n34 = timed-loop {
    timing: w67 -> [_]
    timing-out: [_] -> w66
    tunnel: w40 -> [w349]
    tunnel: [w348] -> w4
    stop <- "E-stop" stop-if-true
    n35 = node-c288() -> (→"E-Stop loop duration (us)":i64)  [unwired: 1 in]
    n36 = xnode "Read/Write Control"("FPGA VI Reference In"=w349) -> ("E-Stop"=w347:bool)  [unwired: 1 in, 2 out]
    "E-Stop" <- w347
    n37 = Or(x=w347, y="E-stop") -> (x .or. y?=w345:bool)
    n38 = node-c288() -> ()  [unwired: 1 in, 1 out]
    n39 = call <vilib>:"Write.vi"("element"=w345) -> ("channel"=w348:T23)  [unwired: 1 out]
  }
  n40 = timed-loop {
    tunnel: [w364] -> w12
    tunnel: w11 -> [w363]
    tunnel: w10 -> [w362]
    tunnel: [w359] -> w9
    timing: w22 -> [_]
    timing-out: [_] -> w21
    tunnel: [w355] -> w5 mode=indexing
    tunnel: w4 -> [w353]
    stop <- w361 stop-if-true
    # "5"
    # "3"
    # "2"
    # "GPS Receive data"
    n41 = node-c288() -> (→"GPS loop duration (us)":i64)  [unwired: 1 in]
    n42 = VISA Read(VISA resource name=w363, byte count=u32 100, error in (no error)=w362) -> (VISA resource name out=w364:refnum<visa-resource-name>, read buffer=w367:string, error out=w360:errorcluster)  [unwired: 1 out]
    n43 = property on="Raw output from GPS" class="Str"(error in=w360, "Text.Scroll Position"=-1 ("Label.Scroll Position")) -> (error out=w359:errorcluster)  [unwired: 1 in, 1 out]
    n44 = feedback #1("") -> (w369:string)
    n45 = Concatenate Strings(w369, w367) -> (w370:string)
    "Raw output from GPS" <- w370
    n46 = feedback-in #1(w370) -> ()
    n47 = while {
      tunnel: [w655] -> w356 mode=indexing
      shift-right: [w654] -> _
      shift-left: w367 -> [w657]
      stop <- w652 stop-if-true
      # "4"
      n48 = Match Pattern(string=w657, regular expression="[, *]") -> (before substring=w655:string, after substring=w654:string, offset past match=w653:i32)  [unwired: 1 in, 1 out]
      n49 = Less Than 0?(x=w653) -> (x < 0?=w652:bool)
    }
    n50 = Index Array(array=w356, index=0) -> (element=w365:string)
    n51 = case shown="\"$GPGSV\"" w365 {
      tunnel: w356 -> [_ w376 w391 w441 w491 w541 w552 w564 w581 w602]
      tunnel: [string[] ["0"] w376 w391 w441 w491 w541 w552 w564 w581 w602] -> w355
      frame "False", Default {
      }
      frame "$GNRMC" {
        n52 = Index Array(array=w376) -> (element #1=→"xxRMC":string, element #2=→"UTC Time":string, element #3=→"Status":string, element #4=→"Lat":string, element #5=→"N/S":string, element #6=→"Long":string, element #7=→"E/W":string, element #8=→"Speed over ground[knot]":string, element #9=→"Course over Ground [Degrees]":string, element #10=→"date[ddmmyy]":string, element #11=→"Mode":string, element #12=→"NavStatus":string, element #13=→"Checksum":string, element #14=→"Carriage return":string)  [unwired: 14 in]
      }
      frame "$GLGSV" {
        n53 = Index Array(array=w391) -> (element #1=→"GLGSV 2":string, element #2=→"number of message 2":string, element #3=w393:string, element #4=→"Satelite in view 2":string)  [unwired: 4 in]
        "msg1 2" <- w393
        n54 = Decimal String To Number(string=w393) -> (number=w392:i32)  [unwired: 2 in, 1 out]
        n55 = case shown="1" w392 {
          tunnel: w391 -> [_ w398 w408 w419 w430]
          frame 0, Default {
          }
          frame 1 {
            n56 = Array Subset(array=w398, index=4) -> (w403:string[])  [unwired: 1 in]
            "Satelite_id/elevation/azimuth/SNR 21" <- w403
            n57 = Array Subset(array=w403, index=4) -> (w404:string[])  [unwired: 1 in]
            "Satelite_id/elevation/azimuth/SNR 20" <- w404
            n58 = Array Subset(array=w404, index=4) -> (w405:string[])  [unwired: 1 in]
            "Satelite_id/elevation/azimuth/SNR 19" <- w405
            n59 = Array Subset(array=w405, index=4) -> (w407:string[])  [unwired: 1 in]
            "Satelite_id/elevation/azimuth/SNR 18" <- w407
            n60 = Array Subset(array=w407, index=4) -> (→"Signal ID / Check sum 5":string[])  [unwired: 1 in]
          }
          frame 2 {
            n61 = Array Subset(array=w408, index=4) -> (w414:string[])  [unwired: 1 in]
            "Satelite_id/elevation/azimuth/SNR 24" <- w414
            n62 = Array Subset(array=w414, index=4) -> (w415:string[])  [unwired: 1 in]
            "Satelite_id/elevation/azimuth/SNR 23" <- w415
            n63 = Array Subset(array=w415, index=4) -> (w416:string[])  [unwired: 1 in]
            "Satelite_id/elevation/azimuth/SNR 22" <- w416
            n64 = Array Subset(array=w416, index=4) -> (w418:string[])  [unwired: 1 in]
            "Satelite_id/elevation/azimuth/SNR 25" <- w418
            n65 = Array Subset(array=w418, index=4) -> (→"Signal ID / Check sum 6":string[])  [unwired: 1 in]
          }
          frame 3 {
            n66 = Array Subset(array=w419, index=4) -> (w425:string[])  [unwired: 1 in]
            "Satelite_id/elevation/azimuth/SNR 28" <- w425
            n67 = Array Subset(array=w425, index=4) -> (w426:string[])  [unwired: 1 in]
            "Satelite_id/elevation/azimuth/SNR 27" <- w426
            n68 = Array Subset(array=w426, index=4) -> (w427:string[])  [unwired: 1 in]
            "Satelite_id/elevation/azimuth/SNR 26" <- w427
            n69 = Array Subset(array=w427, index=4) -> (w429:string[])  [unwired: 1 in]
            "Satelite_id/elevation/azimuth/SNR 29" <- w429
            n70 = Array Subset(array=w429, index=4) -> (→"Signal ID / Check sum 7":string[])  [unwired: 1 in]
          }
          frame 4 {
            n71 = Array Subset(array=w430, index=4) -> (w436:string[])  [unwired: 1 in]
            "Satelite_id/elevation/azimuth/SNR 32" <- w436
            n72 = Array Subset(array=w436, index=4) -> (w437:string[])  [unwired: 1 in]
            "Satelite_id/elevation/azimuth/SNR 31" <- w437
            n73 = Array Subset(array=w437, index=4) -> (w438:string[])  [unwired: 1 in]
            "Satelite_id/elevation/azimuth/SNR 30" <- w438
            n74 = Array Subset(array=w438, index=4) -> (w440:string[])  [unwired: 1 in]
            "Satelite_id/elevation/azimuth/SNR 33" <- w440
            n75 = Array Subset(array=w440, index=4) -> (→"Signal ID / Check sum 8":string[])  [unwired: 1 in]
          }
        }
      }
      frame "$GAGSV" {
        n76 = Index Array(array=w441) -> (element #1=→"GAGSV 3":string, element #2=→"number of message 3":string, element #3=w443:string, element #4=→"Satelite in view 3":string)  [unwired: 4 in]
        "msg1 3" <- w443
        n77 = Decimal String To Number(string=w443) -> (number=w442:i32)  [unwired: 2 in, 1 out]
        n78 = case shown="1" w442 {
          tunnel: w441 -> [_ w448 w458 w469 w480]
          frame 0, Default {
          }
          frame 1 {
            n79 = Array Subset(array=w448, index=4) -> (w453:string[])  [unwired: 1 in]
            "Satelite_id/elevation/azimuth/SNR 38" <- w453
            n80 = Array Subset(array=w453, index=4) -> (w454:string[])  [unwired: 1 in]
            "Satelite_id/elevation/azimuth/SNR 37" <- w454
            n81 = Array Subset(array=w454, index=4) -> (w455:string[])  [unwired: 1 in]
            "Satelite_id/elevation/azimuth/SNR 36" <- w455
            n82 = Array Subset(array=w455, index=4) -> (w457:string[])  [unwired: 1 in]
            "Satelite_id/elevation/azimuth/SNR 35" <- w457
            n83 = Array Subset(array=w457, index=4) -> (→"Signal ID / Check sum 9":string[])  [unwired: 1 in]
          }
          frame 2 {
            n84 = Array Subset(array=w458, index=4) -> (w464:string[])  [unwired: 1 in]
            "Satelite_id/elevation/azimuth/SNR 41" <- w464
            n85 = Array Subset(array=w464, index=4) -> (w465:string[])  [unwired: 1 in]
            "Satelite_id/elevation/azimuth/SNR 40" <- w465
            n86 = Array Subset(array=w465, index=4) -> (w466:string[])  [unwired: 1 in]
            "Satelite_id/elevation/azimuth/SNR 39" <- w466
            n87 = Array Subset(array=w466, index=4) -> (w468:string[])  [unwired: 1 in]
            "Satelite_id/elevation/azimuth/SNR 42" <- w468
            n88 = Array Subset(array=w468, index=4) -> (→"Signal ID / Check sum 10":string[])  [unwired: 1 in]
          }
          frame 3 {
            n89 = Array Subset(array=w469, index=4) -> (w475:string[])  [unwired: 1 in]
            "Satelite_id/elevation/azimuth/SNR 45" <- w475
            n90 = Array Subset(array=w475, index=4) -> (w476:string[])  [unwired: 1 in]
            "Satelite_id/elevation/azimuth/SNR 44" <- w476
            n91 = Array Subset(array=w476, index=4) -> (w477:string[])  [unwired: 1 in]
            "Satelite_id/elevation/azimuth/SNR 43" <- w477
            n92 = Array Subset(array=w477, index=4) -> (w479:string[])  [unwired: 1 in]
            "Satelite_id/elevation/azimuth/SNR 46" <- w479
            n93 = Array Subset(array=w479, index=4) -> (→"Signal ID / Check sum 11":string[])  [unwired: 1 in]
          }
          frame 4 {
            n94 = Array Subset(array=w480, index=4) -> (w486:string[])  [unwired: 1 in]
            "Satelite_id/elevation/azimuth/SNR 49" <- w486
            n95 = Array Subset(array=w486, index=4) -> (w487:string[])  [unwired: 1 in]
            "Satelite_id/elevation/azimuth/SNR 48" <- w487
            n96 = Array Subset(array=w487, index=4) -> (w488:string[])  [unwired: 1 in]
            "Satelite_id/elevation/azimuth/SNR 47" <- w488
            n97 = Array Subset(array=w488, index=4) -> (w490:string[])  [unwired: 1 in]
            "Satelite_id/elevation/azimuth/SNR 50" <- w490
            n98 = Array Subset(array=w490, index=4) -> (→"Signal ID / Check sum 12":string[])  [unwired: 1 in]
          }
        }
      }
      frame "$GBGSV" {
        n99 = Index Array(array=w491) -> (element #1=→"GBGSV 4":string, element #2=→"number of message 4":string, element #3=w493:string, element #4=→"Satelite in view 4":string)  [unwired: 4 in]
        "msg1 4" <- w493
        n100 = Decimal String To Number(string=w493) -> (number=w492:i32)  [unwired: 2 in, 1 out]
        n101 = case shown="1" w492 {
          tunnel: w491 -> [_ w498 w508 w519 w530]
          frame 0, Default {
          }
          frame 1 {
            n102 = Array Subset(array=w498, index=4) -> (w503:string[])  [unwired: 1 in]
            "Satelite_id/elevation/azimuth/SNR 55" <- w503
            n103 = Array Subset(array=w503, index=4) -> (w504:string[])  [unwired: 1 in]
            "Satelite_id/elevation/azimuth/SNR 54" <- w504
            n104 = Array Subset(array=w504, index=4) -> (w505:string[])  [unwired: 1 in]
            "Satelite_id/elevation/azimuth/SNR 53" <- w505
            n105 = Array Subset(array=w505, index=4) -> (w507:string[])  [unwired: 1 in]
            "Satelite_id/elevation/azimuth/SNR 52" <- w507
            n106 = Array Subset(array=w507, index=4) -> (→"Signal ID / Check sum 13":string[])  [unwired: 1 in]
          }
          frame 2 {
            n107 = Array Subset(array=w508, index=4) -> (w514:string[])  [unwired: 1 in]
            "Satelite_id/elevation/azimuth/SNR 58" <- w514
            n108 = Array Subset(array=w514, index=4) -> (w515:string[])  [unwired: 1 in]
            "Satelite_id/elevation/azimuth/SNR 57" <- w515
            n109 = Array Subset(array=w515, index=4) -> (w516:string[])  [unwired: 1 in]
            "Satelite_id/elevation/azimuth/SNR 56" <- w516
            n110 = Array Subset(array=w516, index=4) -> (w518:string[])  [unwired: 1 in]
            "Satelite_id/elevation/azimuth/SNR 59" <- w518
            n111 = Array Subset(array=w518, index=4) -> (→"Signal ID / Check sum 14":string[])  [unwired: 1 in]
          }
          frame 3 {
            n112 = Array Subset(array=w519, index=4) -> (w525:string[])  [unwired: 1 in]
            "Satelite_id/elevation/azimuth/SNR 62" <- w525
            n113 = Array Subset(array=w525, index=4) -> (w526:string[])  [unwired: 1 in]
            "Satelite_id/elevation/azimuth/SNR 61" <- w526
            n114 = Array Subset(array=w526, index=4) -> (w527:string[])  [unwired: 1 in]
            "Satelite_id/elevation/azimuth/SNR 60" <- w527
            n115 = Array Subset(array=w527, index=4) -> (w529:string[])  [unwired: 1 in]
            "Satelite_id/elevation/azimuth/SNR 63" <- w529
            n116 = Array Subset(array=w529, index=4) -> (→"Signal ID / Check sum 15":string[])  [unwired: 1 in]
          }
          frame 4 {
            n117 = Array Subset(array=w530, index=4) -> (w536:string[])  [unwired: 1 in]
            "Satelite_id/elevation/azimuth/SNR 66" <- w536
            n118 = Array Subset(array=w536, index=4) -> (w537:string[])  [unwired: 1 in]
            "Satelite_id/elevation/azimuth/SNR 65" <- w537
            n119 = Array Subset(array=w537, index=4) -> (w538:string[])  [unwired: 1 in]
            "Satelite_id/elevation/azimuth/SNR 64" <- w538
            n120 = Array Subset(array=w538, index=4) -> (w540:string[])  [unwired: 1 in]
            "Satelite_id/elevation/azimuth/SNR 67" <- w540
            n121 = Array Subset(array=w540, index=4) -> (→"Signal ID / Check sum 16":string[])  [unwired: 1 in]
          }
        }
      }
      frame "$GNGLL" {
        n122 = Index Array(array=w541) -> (element #1=→"GLL":string, element #2=→"Lat 2":string, element #3=→"NS":string, element #4=→"Long 3":string, element #5=→"EW":string, element #6=→"Time":string, element #7=→"Status 2":string, element #8=→"Positioning mod":string, element #9=→"Check sum":string, element #10=→"Carriage return 2":string)  [unwired: 10 in]
      }
      frame "$GNVTG" {
        n123 = Index Array(array=w552) -> (element #1=→"VTG":string, element #2=→"Course over Ground":string, element #3=→"Reference":string, element #4=→"Course over Ground (Magnetic)":string, element #5=→"Reference2":string, element #6=→"Speedover Ground (knots)":string, element #7=→"Units1":string, element #8=→"Speed over ground kph":string, element #9=→"Units 2":string, element #10=→"Position Mode 2":string, element #11=→"Check sum 2":string)  [unwired: 11 in]
      }
      frame "$GNGGA" {
        n124 = Index Array(array=w564) -> (element #1=→"GGA 3":string, element #2=→"UTC time":string, element #3=→"Lat 3":string, element #4=→"NS 2":string, element #5=→"Long 2":string, element #6=→"EW 2":string, element #7=→"Pos_indicator":string, element #8=→"Number of Satelite_used":string, element #9=→"hdop":string, element #10=→"msl_altitude":string, element #11=→"altitude_units":string, element #12=→"geoidal_Seperation":string, element #13=→"Separation unit":string, element #14=→"age of Diff corr":string, element #15=→"diffStating":string, element #16=→"Checksum 2":string)  [unwired: 16 in]
      }
      frame "$GNGSA" {
        n125 = Index Array(array=w581) -> (element #1=→"GSA":string, element #2=→"Operation Mode":string, element #3=→"Navigation mode":string, element #4=→"satelite used channel 1":string, element #5=→"satelite used channel 2":string, element #6=→"satelite used channel 3":string, element #7=→"satelite used channel 4":string, element #8=→"satelite used channel 5":string, element #9=→"satelite used channel 6":string, element #10=→"satelite used channel 7":string, element #11=→"satelite used channel 8":string, element #12=→"satelite used channel 9":string, element #13=→"satelite used channel 10":string, element #14=→"satelite used channel 11":string, element #15=→"satelite used channel 12":string, element #16=→"pdop":string, element #17=→"hdop 2":string, element #18=→"vdop":string, element #19=→"System ID":string, element #20=→"Checksum 3":string)  [unwired: 20 in]
      }
      frame "$GPGSV" {
        n126 = Index Array(array=w602) -> (element #1=→"GPGSV":string, element #2=→"number of message":string, element #3=w604:string, element #4=→"Satelite in view":string)  [unwired: 4 in]
        "msg1" <- w604
        n127 = Decimal String To Number(string=w604) -> (number=w603:i32)  [unwired: 2 in, 1 out]
        n128 = case shown="1" w603 {
          tunnel: w602 -> [_ w609 w619 w630 w641]
          frame 0, Default {
          }
          frame 1 {
            n129 = Array Subset(array=w609, index=4) -> (w614:string[])  [unwired: 1 in]
            "Satelite_id/elevation/azimuth/SNR" <- w614
            n130 = Array Subset(array=w614, index=4) -> (w615:string[])  [unwired: 1 in]
            "Satelite_id/elevation/azimuth/SNR 2" <- w615
            n131 = Array Subset(array=w615, index=4) -> (w616:string[])  [unwired: 1 in]
            "Satelite_id/elevation/azimuth/SNR 3" <- w616
            n132 = Array Subset(array=w616, index=4) -> (w618:string[])  [unwired: 1 in]
            "Satelite_id/elevation/azimuth/SNR 4" <- w618
            n133 = Array Subset(array=w618, index=4) -> (→"Signal ID / Check sum":string[])  [unwired: 1 in]
          }
          frame 2 {
            n134 = Array Subset(array=w619, index=4) -> (w625:string[])  [unwired: 1 in]
            "Satelite_id/elevation/azimuth/SNR 5" <- w625
            n135 = Array Subset(array=w625, index=4) -> (w626:string[])  [unwired: 1 in]
            "Satelite_id/elevation/azimuth/SNR 6" <- w626
            n136 = Array Subset(array=w626, index=4) -> (w627:string[])  [unwired: 1 in]
            "Satelite_id/elevation/azimuth/SNR 7" <- w627
            n137 = Array Subset(array=w627, index=4) -> (w629:string[])  [unwired: 1 in]
            "Satelite_id/elevation/azimuth/SNR 8" <- w629
            n138 = Array Subset(array=w629, index=4) -> (→"Signal ID / Check sum 2":string[])  [unwired: 1 in]
          }
          frame 3 {
            n139 = Array Subset(array=w630, index=4) -> (w636:string[])  [unwired: 1 in]
            "Satelite_id/elevation/azimuth/SNR 9" <- w636
            n140 = Array Subset(array=w636, index=4) -> (w637:string[])  [unwired: 1 in]
            "Satelite_id/elevation/azimuth/SNR 10" <- w637
            n141 = Array Subset(array=w637, index=4) -> (w638:string[])  [unwired: 1 in]
            "Satelite_id/elevation/azimuth/SNR 11" <- w638
            n142 = Array Subset(array=w638, index=4) -> (w640:string[])  [unwired: 1 in]
            "Satelite_id/elevation/azimuth/SNR 12" <- w640
            n143 = Array Subset(array=w640, index=4) -> (→"Signal ID / Check sum 3":string[])  [unwired: 1 in]
          }
          frame 4 {
            n144 = Array Subset(array=w641, index=4) -> (w647:string[])  [unwired: 1 in]
            "Satelite_id/elevation/azimuth/SNR 13" <- w647
            n145 = Array Subset(array=w647, index=4) -> (w648:string[])  [unwired: 1 in]
            "Satelite_id/elevation/azimuth/SNR 14" <- w648
            n146 = Array Subset(array=w648, index=4) -> (w649:string[])  [unwired: 1 in]
            "Satelite_id/elevation/azimuth/SNR 15" <- w649
            n147 = Array Subset(array=w649, index=4) -> (w651:string[])  [unwired: 1 in]
            "Satelite_id/elevation/azimuth/SNR 16" <- w651
            n148 = Array Subset(array=w651, index=4) -> (→"Signal ID / Check sum 4":string[])  [unwired: 1 in]
          }
        }
      }
    }
    n149 = call <extravilib>:"Read.vi"("channel"=w353) -> ("element"=w354:bool)  [unwired: 1 in, 1 out]
    n150 = Or(x=w359, y=w354) -> (x .or. y?=w361:bool)
    n151 = node-c288() -> ()  [unwired: 1 in, 1 out]
  }
  n152 = timed-loop {
    timing: w71 -> [_]
    timing-out: [_] -> w70
    tunnel: w40 -> [w670]
    tunnel: [w669] -> w26
    tunnel: w4 -> [w663]
    tunnel: w6 -> [_]
    tunnel: [w658] -> w28 mode=indexing
    stop <- w664 stop-if-true
    n153 = node-c288() -> (→"Encoder data gathering duration(us)":i64)  [unwired: 1 in]
    n154 = xnode "Read/Write Control"("FPGA VI Reference In"=w670, "Position Reset"="Encoder Position Reset", "Velocity Interval (uSec)"=u32 1000) -> ("error out"=w669:errorcluster, "Position (Counts)"=w661:i32, "Acceleration (Counts/Interval)"=w660:i32, "Velocity (Counts/Interval)"=w659:i32)  [unwired: 1 in, 1 out]
    "Encoder Position (Counts)" <- w661
    "Encoder Acceleration (Counts/Interval)" <- w660
    "Encoder Velocity (Counts/Interval)" <- w659
    n155 = Build Array(w661, w660, w659) -> (w658:i32[])
    n156 = call <extravilib>:"Read.vi"("channel"=w663) -> ("element"=w666:bool)  [unwired: 1 in, 1 out]
    n157 = node-c288() -> ()  [unwired: 1 in, 1 out]
    n158 = Or(x=w666, y="Encoder") -> (x .or. y?=w664:bool)
  }
  n159 = timed-loop {
    timing: w69 -> [_]
    timing-out: [_] -> w68
    tunnel: [w695] -> w57
    tunnel: [w696] -> w56
    tunnel: [w697] -> w55
    tunnel: w32 -> [w735]
    tunnel: [w694] -> w54
    tunnel: [w693] -> w53
    tunnel: w33 -> [w674]
    shift-right: [w692] -> w52
    shift-left: w8 -> [w734]
    tunnel: w4 -> [w688]
    tunnel: w6 -> [_]
    tunnel: [w675] -> w29 mode=indexing
    tunnel: [w674] -> w7
    stop <- w691 stop-if-true
    w702 = u32 2 ("Byte Count")
    w718 = u32 2 ("Byte Count")
    n160 = node-c288() -> (→"IMU Data gathering duration(us)":i64)  [unwired: 1 in]
    n161 = call <vilib>:"Write Read.vi"("Byte Count"=w718, "error in (no error)"=w734, "Bytes to Write"=u8[] [44], "Slave Address (7-bit)"=w735, "I2C Ref In"=w674) -> ("error out"=w695:errorcluster, "Bytes Read"=w726:u8[])  [unwired: 3 in, 1 out]
    n162 = call <vilib>:"Write Read.vi"("Byte Count"=w718, "error in (no error)"=w734, "Bytes to Write"=u8[] [42], "Slave Address (7-bit)"=w735, "I2C Ref In"=w674) -> ("error out"=w696:errorcluster, "Bytes Read"=w728:u8[])  [unwired: 3 in, 1 out]
    n163 = call <vilib>:"Write Read.vi"("Byte Count"=w718, "error in (no error)"=w734, "Bytes to Write"=u8[] [40], "Slave Address (7-bit)"=w735, "I2C Ref In"=w674) -> ("error out"=w697:errorcluster, "Bytes Read"=w730:u8[])  [unwired: 3 in, 1 out]
    n164 = call <vilib>:"Write Read.vi"("Byte Count"=w702, "error in (no error)"=w734, "Bytes to Write"=u8[] [28], "Slave Address (7-bit)"=w735, "I2C Ref In"=w674) -> ("error out"=w692:errorcluster, "Bytes Read"=w710:u8[])  [unwired: 3 in, 1 out]
    n165 = call <vilib>:"Write Read.vi"("Byte Count"=w702, "error in (no error)"=w734, "Bytes to Write"=u8[] [26], "Slave Address (7-bit)"=w735, "I2C Ref In"=w674) -> ("error out"=w693:errorcluster, "Bytes Read"=w712:u8[])  [unwired: 3 in, 1 out]
    n166 = call <vilib>:"Write Read.vi"("Byte Count"=w702, "error in (no error)"=w734, "Bytes to Write"=u8[] [24], "Slave Address (7-bit)"=w735, "I2C Ref In"=w674) -> ("error out"=w694:errorcluster, "Bytes Read"=w714:u8[])  [unwired: 3 in, 1 out]
    n167 = Index Array "Index Array"(array=w710) -> (element #1=w708:u8, element #2=w707:u8)  [unwired: 2 in]
    n168 = Index Array "Index Array"(array=w712) -> (element #1=w706:u8, element #2=w705:u8)  [unwired: 2 in]
    n169 = Index Array "Index Array"(array=w728) -> (element #1=w722:u8, element #2=w721:u8)  [unwired: 2 in]
    n170 = Index Array "Index Array"(array=w730) -> (element #1=w720:u8, element #2=w719:u8)  [unwired: 2 in]
    n171 = Index Array "Index Array"(array=w726) -> (element #1=w724:u8, element #2=w723:u8)  [unwired: 2 in]
    n172 = Index Array "Index Array"(array=w714) -> (element #1=w704:u8, element #2=w703:u8)  [unwired: 2 in]
    n173 = Join Numbers(hi=w723, lo=w724) -> ((hi.lo)=w733:u16)
    n174 = Join Numbers(hi=w721, lo=w722) -> ((hi.lo)=w732:u16)
    n175 = Join Numbers(hi=w719, lo=w720) -> ((hi.lo)=w731:u16)
    n176 = Join Numbers(hi=w707, lo=w708) -> ((hi.lo)=w717:u16)
    n177 = Join Numbers(hi=w705, lo=w706) -> ((hi.lo)=w716:u16)
    n178 = Join Numbers(hi=w703, lo=w704) -> ((hi.lo)=w715:u16)
    n179 = To Word Integer(number=w733) -> (16bit integer=w681:i16)
    n180 = To Word Integer(number=w732) -> (16bit integer=w682:i16)
    n181 = To Word Integer(number=w731) -> (16bit integer=w683:i16)
    n182 = To Word Integer(number=w717) -> (16bit integer=w686:i16)
    n183 = To Word Integer(number=w716) -> (16bit integer=w685:i16)
    n184 = To Word Integer(number=w715) -> (16bit integer=w684:i16)
    n185 = Bundle "Bundle"(w686, w685, w684) -> (w699:cluster{i16, i16, i16})  [unwired: 1 in]
    n186 = Bundle "Bundle"(w681, w682, w683) -> (w700:cluster{i16, i16, i16})  [unwired: 1 in]
    n187 = Multiply(x=w699, y=0.0175) -> (x*y=w680:cluster{dbl, dbl, dbl})
    "IMU Gyro Chart" <- w680
    n188 = Multiply(x=w700, y=0.000122) -> (x*y=w679:cluster{dbl, dbl, dbl})
    "IMU Acc Chart" <- w679
    n189 = Cluster To Array(cluster=w679) -> (array=w677:dbl[])
    n190 = Cluster To Array(cluster=w680) -> (array=w678:dbl[])
    n191 = call <extravilib>:"Read.vi"("channel"=w688) -> ("element"=w689:bool)  [unwired: 1 in, 1 out]
    n192 = Or(x=w689, y="IMU") -> (x .or. y?=w691:bool)
    n193 = Insert Into Array(array=w678, index=3, new element=w677) -> (w675:dbl[])
    n194 = node-c288() -> ()  [unwired: 1 in, 1 out]
  }
  n195 = timed-loop {
    tunnel: w61 -> [w749]
    tunnel: w40 -> [w748]
    tunnel: [w747] -> w58
    tunnel: [w746] -> w24
    timing: w73 -> [_]
    timing-out: [_] -> w72
    tunnel: w4 -> [w741]
    tunnel: w6 -> [_]
    tunnel: [w739] -> w27 mode=indexing
    stop <- w742 stop-if-true
    n196 = node-c288() -> (→"Hall data gathering duration(us)":i64)  [unwired: 1 in]
    n197 = xnode "Read/Write Control"("FPGA VI Reference In"=w748, "error in"=w749) -> ("FPGA VI Reference Out"=w747:refnum<k20>, "error out"=w746:errorcluster, "Hall Period"=w739:u32, "Hall Detection"=→"Hall Detection":bool)
    "Hall Period" <- w739
    n198 = call <extravilib>:"Read.vi"("channel"=w741) -> ("element"=w743:bool)  [unwired: 1 in, 1 out]
    n199 = node-c288() -> ()  [unwired: 1 in, 1 out]
    n200 = Or(x=w743, y="Hall") -> (x .or. y?=w742:bool)
  }
  n201 = for {
    tunnel: w6 -> [w755]
    tunnel: w5 -> [w754] mode=indexing
    tunnel: [w753] -> w1 mode=indexing
    n202 = TDMS Write(0:w755, 1:enum16{"decimated", "interleaved"}."interleaved" ("data layout (0:decimated)"), 5:"GPS" ("group name in (Untitled)"), 9:w754) -> (15:w753:errorcluster)  [unwired: 2 in, 3 out]
  }
  n203 = node-c288(w66) -> (w39:i64)
  n204 = node-c288(w72) -> (w38:i64)
  n205 = node-c288(w70) -> (w37:i64)
  n206 = for {
    tunnel: w6 -> [w761]
    tunnel: w28 -> [w760] mode=indexing
    tunnel: w26 -> [w759]
    tunnel: [w758] -> w25 mode=indexing
    n207 = TDMS Write(0:w761, 1:enum16{"decimated", "interleaved"}."interleaved" ("data layout (0:decimated)"), 5:"Encoder" ("group name in (Untitled)"), 7:string[] ["Position", "Acc", "Velocity"] ("channel name(s) in (Untitled)"), 9:w760, 11:w759) -> (15:w758:errorcluster)  [unwired: 3 out]
  }
  n208 = for {
    tunnel: w6 -> [w769]
    tunnel: w27 -> [w767] mode=indexing
    tunnel: w24 -> [w766]
    tunnel: [w765] -> w23 mode=indexing
    n209 = Build Array(w767) -> (w768:u32[])
    n210 = TDMS Write(0:w769, 5:"Hall" ("group name in (Untitled)"), 7:string[] ["Period"] ("channel name(s) in (Untitled)"), 9:w768, 11:w766) -> (15:w765:errorcluster)  [unwired: 1 in, 3 out]
  }
  n211 = node-c288(w68) -> (w35:i64)
  n212 = call <vilib>:"Close.vi"("I2C Ref In"=w7) -> ()  [unwired: 10 in, 1 out]
  n213 = Merge Errors(w52, w53, w54, w57, w56, w55) -> (w43:errorcluster)
  n214 = node-c288(w21) -> ()  [unwired: 1 out]
  n215 = VISA Flush I/O Buffer(VISA resource name=w12, error in (no error)=w9) -> (VISA resource name out=w14:refnum<visa-resource-name>, error out=w13:errorcluster)  [unwired: 1 in]
  n216 = for {
    tunnel: [w774] -> w30 mode=indexing
    tunnel: w6 -> [w773]
    tunnel: w29 -> [w772] mode=indexing
    n217 = TDMS Write(0:w773, 1:enum16{"decimated", "interleaved"}."interleaved" ("data layout (0:decimated)"), 5:"IMU" ("group name in (Untitled)"), 7:string[] ["Gyro X", "Gyro Y", "Gyro Z", "Acc X", "Acc Y", "Acc Z"] ("channel name(s) in (Untitled)"), 9:w772) -> (15:w774:errorcluster)  [unwired: 1 in, 3 out]
  }
  n218 = VISA Close(VISA resource name=w14, error in (no error)=w13) -> (error out=w3:errorcluster)
  n219 = Compound Arithmetic op=ADD(w39, w38, w37, w35, w36) -> (→"Combined duration time (us)":i64)
  n220 = Merge Errors(w3, w1) -> (w2:errorcluster)
  n221 = Merge Errors(w23, w25, w43, w30, w2) -> (w42:errorcluster)
  n222 = call <vilib>:"Simple Error Handler.vi"("error in (no error)"=w42) -> ("error out"=w41:errorcluster)  [unwired: 4 in, 4 out]
  n223 = xnode "Invoke Method"("FPGA VI Reference In"=w58, "error in"=w41) -> ("FPGA VI Reference Out"=w60:refnum<k20>, "error out"=w31:errorcluster)
  n224 = call <vilib>:"Reset myRIO.vi"("error in (no error)"=w31) -> ("error out"=w59:errorcluster)  [unwired: 10 in]
  n225 = TDMS Close(8:w31, 11:w6) -> ()  [unwired: 2 out]
  n226 = xnode "Close FPGA VI Reference"("FPGA VI Reference In"=w60, "error in"=w59) -> ()  [unwired: 1 out]
